vi "Cap Probe FPGA Voltage to Displacement.vi"(9 "Micrometers per Volt":dbl, 11 "Cap Probe FPGA Voltage":u16) -> (3 "Cap Probe Displacement":dbl)   [LabVIEW 2018]
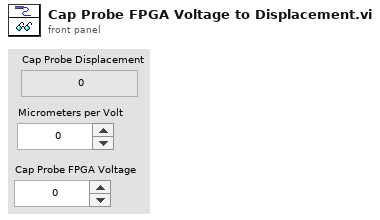
[diagram p1: front panel]
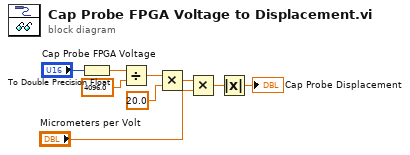
[diagram p0: block diagram]
diagram:
  n1 = To Double Precision Float(number="Cap Probe FPGA Voltage") -> (double precision float=w9:dbl)
  n2 = Divide(x=w9, y=4096.0) -> (x/y=w7:dbl)
  n3 = Multiply(x=w7, y=20.0) -> (x*y=w5:dbl)
  n4 = Multiply(x=w5, y="Micrometers per Volt") -> (x*y=w2:dbl)
  n5 = Absolute Value(x=w2) -> (abs(x)=→"Cap Probe Displacement":dbl)
